vi "Logout.vi"(8 "error in (no error)":errorcluster, 11 "Session in":refnum<class "Session.lvclass">) -> (0 "error out":errorcluster, 3 "Session out":refnum<class "Session.lvclass">)   [LabVIEW 2016, in "Session.lvclass"]
uses:
  Session.lvclass
  Session.lvclass/Session.ctl
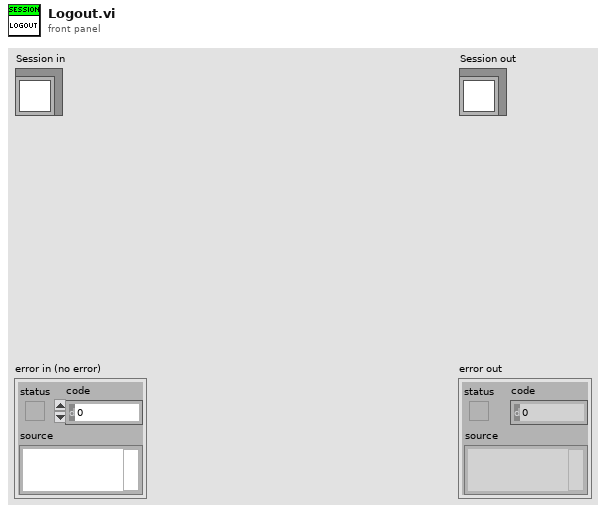
[diagram p1: front panel]
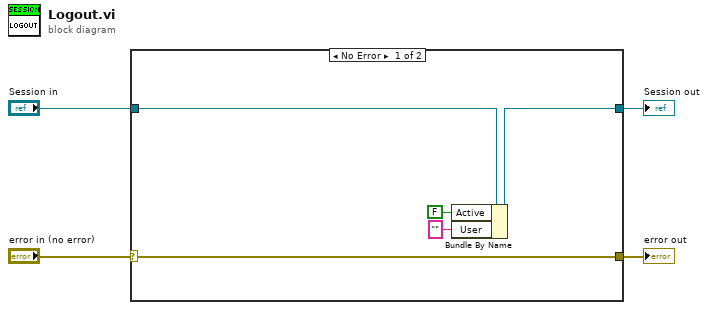
[diagram p0: block diagram]
diagram:
  n1 = case shown="No Error" "error in (no error)" {
    selector: "error in (no error)" -> [w7 w11]
    tunnel: [w7 w11] -> w3
    tunnel: [w8 w10] -> w1
    tunnel: "Session in" -> [w9 w10]
    frame No Error {
      n2 = Bundle By Name(cluster=w9, "Active"=FALSE, "User"="") -> (w8:refnum<class "Session.lvclass">)
    }
    frame Error {
    }
  }
  "error out" <- w3
  "Session out" <- w1
